vi "writeToXML.vi"(8 "error in (no error)":errorcluster, 10 "ClassLabel":string, 11 "POffset in":refnum<class "POffset.lvclass">) -> (0 "error out":errorcluster, 2 "XML out":string, 3 "POffset out":refnum<class "POffset.lvclass">)   [LabVIEW 2022 SP3, in "TCSDataDefinitions.lvlib" / "TCSCommand.lvlib" / "POriginCommands.lvlib" / "POffset.lvclass"]
uses:
  POffset.lvclass
  <userlib>/Common/UnitsAndXML/FlattenItemWithUnitToXML/FlattenLengthToXML/LengthUnit.ctl
  POffset.lvclass/POffset.ctl
  POriginCommands/POriginCommands.lvclass
  <userlib>/Common/UnitsAndXML/UnitsAndXML.lvlib
  <userlib>/Common/XML/XMLGenerator/XMLGenerator.lvclass
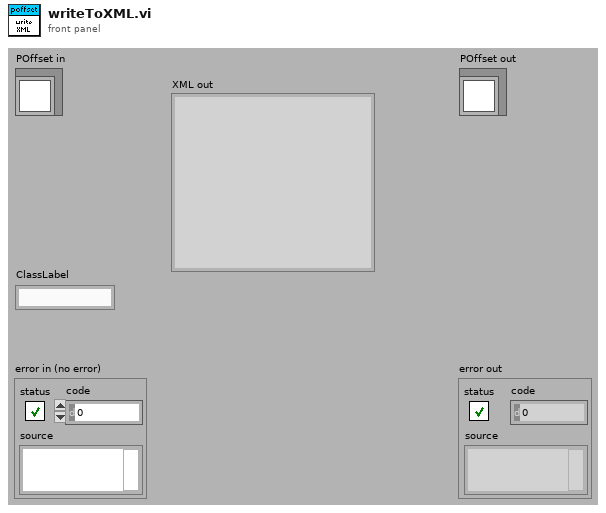
[diagram p1: front panel]
types:
  T1 = typedef "UnitsAndXML.lvlib/LengthUnit.ctl" = enum16{"m", "Angstrom", "AU", "chain", "cm", "cubit", "fathom", "fermi", "ft", "furlong", "hubble", "in", "ly", "mi", "mm", "rod", "um", "yd"}
  T2 = typedef "TCSDataDefinitions.lvlib/TCSCommand.lvlib/OffsetCommands.lvlib/Num1Types.ctl" = enum16{"User", "Handset"}
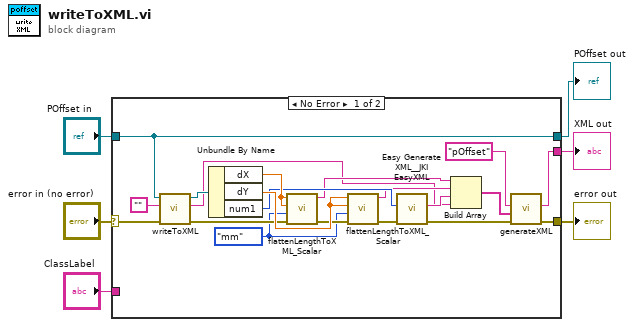
[diagram p0: block diagram]
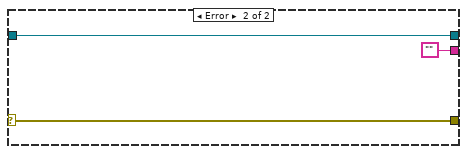
[diagram p2: hidden frame]
diagram:
  n1 = case shown="No Error" "error in (no error)" {
    selector: "error in (no error)" -> [w16 w29]
    tunnel: [w9 w29] -> w5
    tunnel: [w19 w28] -> w3
    tunnel: "POffset in" -> [w19 w28]
    tunnel: [w8 ""] -> w2
    tunnel: "ClassLabel" -> [_ _]
    frame No Error {
      w7 = LengthUnit."mm" ("lengthUnitInXML")
      n2 = call-parent "writeToXML.vi"("error in (no error)"=w16, "ClassLabel"="", "POriginCommands in"=w19) -> ("error out"=w15:errorcluster, "XML out"=w13:string, "POriginCommands out"=w18:refnum<class "POffset.lvclass">)  [unwired: 6 in]
      n3 = Unbundle By Name(w18) -> ("dX"=w26:dbl[unit], "dY"=w25:dbl[unit], "num1"=w24:T2)
      n4 = call <userlib>:"flattenLengthToXML_Scalar.vi"("error in (no error)"=w15, "lengthUnitInXML"=w7, "lengthAgain"=w26, "length"=w26) -> ("error out"=w23:errorcluster, "xmlString"=w21:string)  [unwired: 6 in]
      n5 = call <userlib>:"flattenLengthToXML_Scalar.vi"("error in (no error)"=w23, "lengthUnitInXML"=w7, "lengthAgain"=w25, "length"=w25) -> ("error out"=w22:errorcluster, "xmlString"=w20:string)  [unwired: 6 in]
      n6 = call <vilib>:"Easy Generate XML__JKI EasyXML.vi"("error in (no error)"=w22, "LabVIEW Data"=w24) -> ("error out"=w10:errorcluster, "XML String"=w14:string)  [unwired: 8 in]
      n7 = Build Array(w21, w20, w14, w13) -> (w12:string[])
      n8 = call <userlib>:"generateXML.vi"("error in"=w10, "childrenXML"=w12, "elementName"="pOffset" ("Class Label")) -> ("error out"=w9:errorcluster, "XML out"=w8:string)  [unwired: 6 in, 1 out]
    }
    frame Error {
    }
  }
  "error out" <- w5
  "POffset out" <- w3
  "XML out" <- w2
